vi "ConvertedFileDialogSubVI.vi"(0 "start path":path=path "", 1 "prompt":string, 3 "button label":string, 7 "default name":string, 11 "error in":errorcluster, 12 "pattern (all files)":string, 14 "pattern label":string) -> (4 "selected path":path, 8 "exists":bool, 10 "cancelled":bool, 15 "error out":errorcluster)   [LabVIEW 2011]
doc: "Displays a dialog box with which you can specify the path to a file or directory.\n--------------------\n\nThis Express VI is configured as follows:\n\nSelection Mode: \nNew or existing file"
panel:
  out "selected paths":path[](array[path])
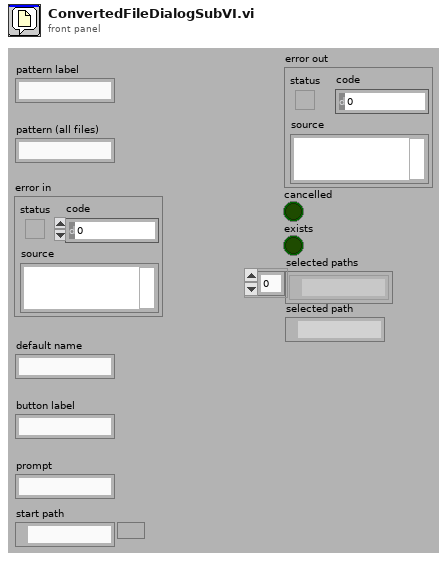
[diagram p1: front panel]
types:
  T1 = enum32{"existing file", "new file", "new or existing file", "existing dir", "new dir", "new or existing dir", "existing file (use LLBs)", "new file (use LLBs)", "new or existing file (use LLBs)", "new or existing file or directory (use LLBs)", "existing dir (use LLBs)", "new dir (use LLBs)", "new or existing dir (use LLBs)", "existing file or dir", "new file or dir", "new or existing file or dir", "existing file or dir (use LLBs)", "new file or dir (use LLBs)", "multi-select", "multi-select (use LLBs)"}
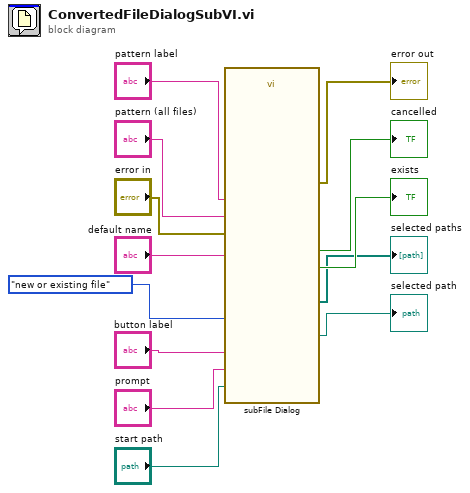
[diagram p0: block diagram]
diagram:
  n1 = call <vilib>:"subFile Dialog.vi"("start path"="start path", "prompt"="prompt", "button label"="button label", "selection mode"=T1."new or existing file", "default name"="default name", "error in"="error in", "pattern (all files)"="pattern (all files)", "pattern label"="pattern label") -> ("selected path"=→"selected path":path, "selected paths"=→"selected paths":path[], "exists"=→"exists":bool, "cancelled"=→"cancelled":bool, "error out"=→"error out":errorcluster)  [unwired: 3 in]
